vi "Fix gRPC Server Dependencies.vi"(8 "error in":errorcluster, 9 "Proto Names":T1, 10 "Project Path":path, 11 "VI Refnum":refnum<vi>) -> (0 "error out":errorcluster)   [LabVIEW 2021, in "Plugin Generator.lvlib"]
uses:
  Plugin Generator.lvlib
  Typedef/Proto Names.ctl
  <vilib>/Utility/traverseref.llb/TRef TravTarget.ctl
  <vilib>/Utility/traverseref.llb/VI Scripting - Traverse.lvlib
  <vilib>/CIF Foundation/CIF LabVIEW Scripting/LV Scripting/LV Scripting Utilities.lvlib
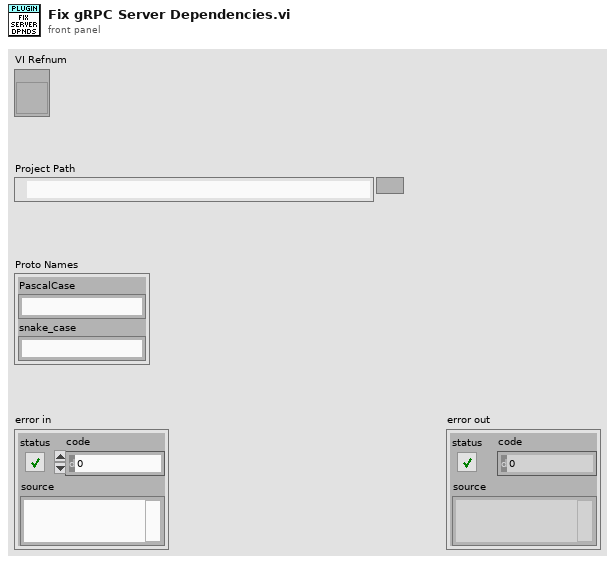
[diagram p1: front panel]
types:
  T1 = typedef "Plugin Generator.lvlib/Proto Names.ctl" = cluster{"PascalCase":string, "snake_case":string}
  T2 = typedef "TRef TravTarget.ctl" = enum16{"FP", "BD", "Other"}
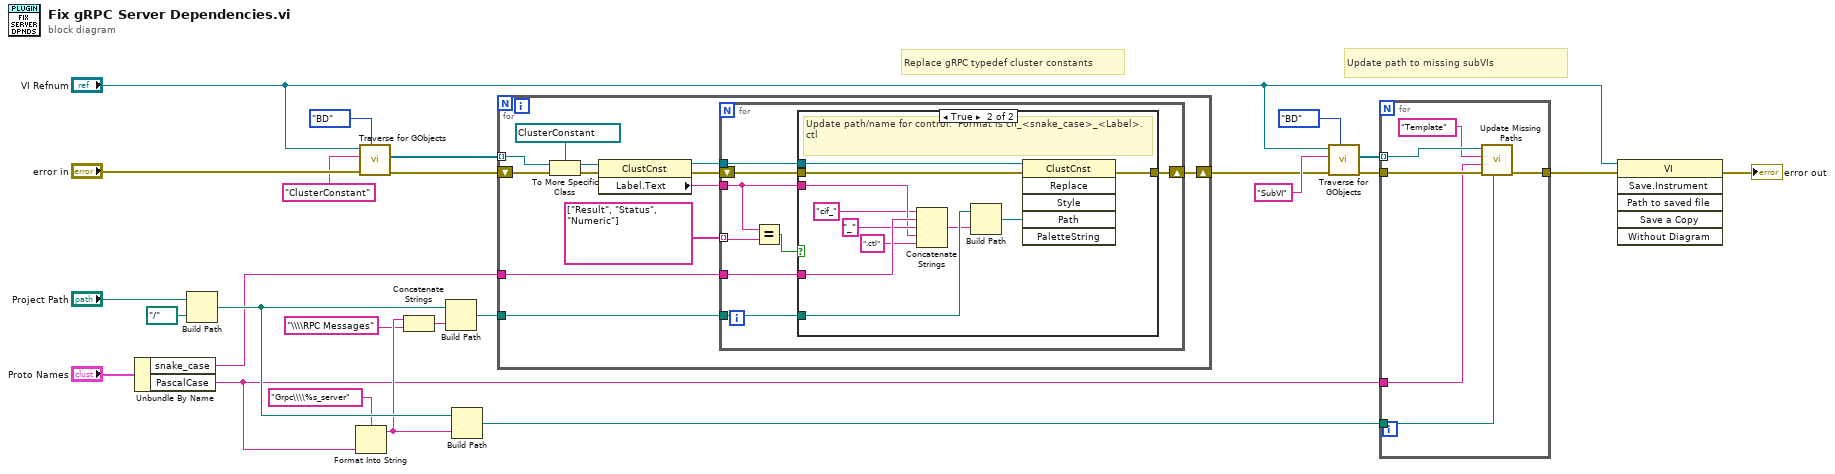
[diagram p0: block diagram]
diagram:
  # "Update path to missing subVIs"
  # "Replace gRPC typedef cluster constants"
  n1 = Unbundle By Name("Proto Names") -> ("snake_case"=w14:string, "PascalCase"=w2:string)
  n2 = Build Path(base path="Project Path", name or relative path=path "../..") -> (appended path=w15:path)
  n3 = Format Into String(format string="Grpc\\\\%s_server" ("Class Name"), w2) -> (resulting string=w12:string)  [unwired: 2 in, 1 out]
  n4 = call <vilib>:"Traverse for GObjects.vi"("Traverse Target"=TRef_TravTarget."BD", "error in (no error)"="error in", "Class Name"="ClusterConstant", "VI Refnum"="VI Refnum") -> ("error out"=w17:errorcluster, "References"=w21:refnum<vi>[])  [unwired: 4 in, 2 out]
  n5 = Concatenate Strings(w12, "\\\\RPC Messages" ("Class Name")) -> (w10:string)
  n6 = Build Path(base path=w15, name or relative path=w10) -> (appended path=w16:path)
  n7 = Build Path(base path=w15, name or relative path=w12) -> (appended path=w1:path)
  n8 = for {
    tunnel: w21 -> [w37] mode=indexing
    tunnel: w14 -> [w30]
    shift-right: [w32] -> w4
    shift-left: w17 -> [w28]
    tunnel: w16 -> [w27]
    n9 = To More Specific Class(target class=refnum<vi> refnum ("x"), reference=w37, error in=w28) -> (specific class reference=w31:refnum<vi>, error out=w35:errorcluster)
    n10 = property class="ClustCnst"(reference=w31, error in=w35) -> (reference out=w33:refnum<vi>, error out=w34:errorcluster, "Label.Text"=w29:string)
    n11 = for {
      tunnel: w33 -> [w44]
      tunnel: w30 -> [w41]
      tunnel: w29 -> [w38]
      tunnel: w27 -> [w42]
      shift-right: [w43] -> w32
      shift-left: w34 -> [w45]
      tunnel: string[] ["Result", "Status", "Numeric"] -> [w40] mode=indexing
      n12 = Equal?(x=w38, y=w40) -> (x = y?=w39:bool)
      n13 = case shown="True" w39 {
        tunnel: w45 -> [w46 w51]
        tunnel: w44 -> [_ w57]
        tunnel: [w46 w56] -> w43
        tunnel: w42 -> [_ w55]
        tunnel: w41 -> [_ w53]
        tunnel: w38 -> [_ w50]
        frame False {
        }
        frame True {
          # "Update path/name for control.  Format is cif_<snake_case>_<Label>.ctl"
          n14 = Concatenate Strings("cif_", w53, "_" ("string"), w50, ".ctl" ("string")) -> (w48:string)
          n15 = Build Path(base path=w55, name or relative path=w48) -> (appended path=w54:path)
          n16 = invoke class="ClustCnst" method="Replace"(reference=w57, error in=w51, "Path"=w54) -> (error out=w56:errorcluster)  [unwired: 3 in, 5 out]
        }
      }
    }
  }
  n17 = call <vilib>:"Traverse for GObjects.vi"("Traverse Target"=TRef_TravTarget."BD", "error in (no error)"=w4, "Class Name"="SubVI", "VI Refnum"="VI Refnum") -> ("error out"=w6:errorcluster, "References"=w7:refnum<vi>[])  [unwired: 4 in, 2 out]
  n18 = for {
    tunnel: w7 -> [w62] mode=indexing
    tunnel: w2 -> [w61]
    tunnel: w6 -> [w63]
    tunnel: [w60] -> w3
    tunnel: w1 -> [w59]
    n19 = call <vilib>:"Update Missing Paths.vi"("Search Path"=w59, "error in (no error)"=w63, "New Subname"=w61, "Subname to Replace"="Template" ("search string"), "GObject in"=w62) -> ("error out"=w60:errorcluster)  [unwired: 6 in]
  }
  n20 = invoke class="VI" method="Save.Instrument"(reference="VI Refnum", error in=w3) -> (error out=→"error out":errorcluster)  [unwired: 4 in, 5 out]
